vi "RT Global.vi"() -> ()   [LabVIEW 2022 SP3]
panel:
  in  "Seq State":string
  out "Abort Seq":bool
  in  "AO CN":string[](array[string])
  in  "DO CN":string[](array[string])
  out "Ready For Seq":bool
  in  "AO task":refnum<k21>
  out "DO task":refnum<k21>
  out "Start DAQ":bool
  out "Connected?":bool
  out "RT Exit":bool
  in  "reader url":refnum<k21>
  in  "Writer URL":refnum<k21>
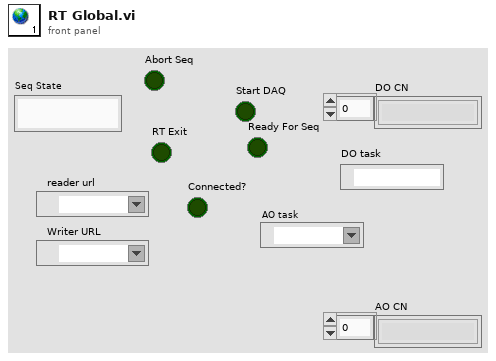
[diagram p1: front panel]
diagram:
